vi "Acquisition Stoped.vi"(8 "error in (no error)":errorcluster, 11 "HIJ Vision Display in":refnum<class "HIJ Vision Display.lvclass">) -> (0 "error out":errorcluster, 3 "HIJ Vision Display out":refnum<class "HIJ Vision Display.lvclass">)   [LabVIEW 2020, in "HIJ Vision Display.lvlib" / "HIJ Vision Display.lvclass"]
uses:
  HIJ Vision Display.lvclass
  HIJ Vision Display.lvclass/HIJ Vision Display.ctl
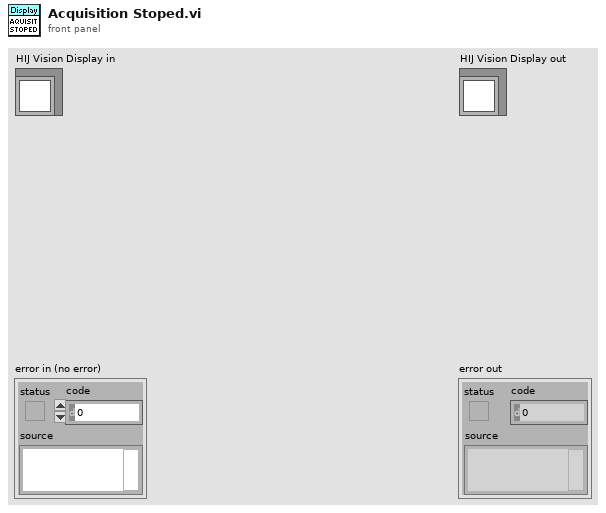
[diagram p1: front panel]
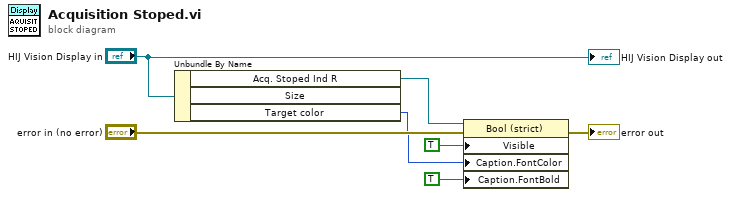
[diagram p0: block diagram]
diagram:
  n1 = Unbundle By Name("HIJ Vision Display in") -> ("Acq. Stoped Ind R"=w6:refnum<vi>, "Target color"=w2:u32)  [unwired: 1 out]
  n2 = property class="Bool (strict)"(reference=w6, error in="error in (no error)", "Visible"=TRUE, "Caption.FontColor"=w2, "Caption.FontBold"=TRUE ("Label.Font:Bold")) -> (error out=→"error out":errorcluster)  [unwired: 1 out]
  "HIJ Vision Display out" <- "HIJ Vision Display in"
